vi "Read.vi"(11 "OutOfRange Condition Config in":refnum<class "OutOfRange Condition Config.lvclass">) -> (1 "Low Limit":dbl, 2 "High Limit":dbl, 3 "Source":string)   [LabVIEW 2020, in "VolatusSeqConfig.lvlib" / "OutOfRange Condition Config.lvclass"]
uses:
  OutOfRange Condition Config.lvclass
  OutOfRange Condition Config.lvclass/OutOfRange Condition Config.ctl
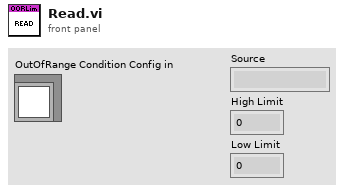
[diagram p1: front panel]
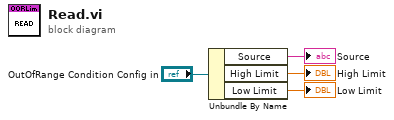
[diagram p0: block diagram]
diagram:
  n1 = Unbundle By Name("OutOfRange Condition Config in") -> ("Source"=→"Source":string, "High Limit"=→"High Limit":dbl, "Low Limit"=→"Low Limit":dbl)
